vi "Create Dir in FTP if Not Exist.vi"(8 "error in (no error)":errorcluster, 10 "dir":string, 11 "FTPProtocol in":refnum<class "FTPProtocol.lvclass">) -> (0 "error out":errorcluster, 3 "FTPProtocol out":refnum<class "FTPProtocol.lvclass">)   [LabVIEW 2020, in "CSM-FileSync.lvlib" / "FTPProtocol.lvclass"]
uses:
  FTPProtocol.lvclass
  FTPProtocol.lvclass/FTPProtocol.ctl
  Read FTP.vi
  FTP Toolkit/FTP Class/FTP.lvclass
  <userlib>/_NEVSTOP/Communicable State Machine(CSM)/_Shared/CSM Shared.lvlib
  <userlib>/_NEVSTOP/Communicable State Machine(CSM)/Communicable State Machine.lvlib
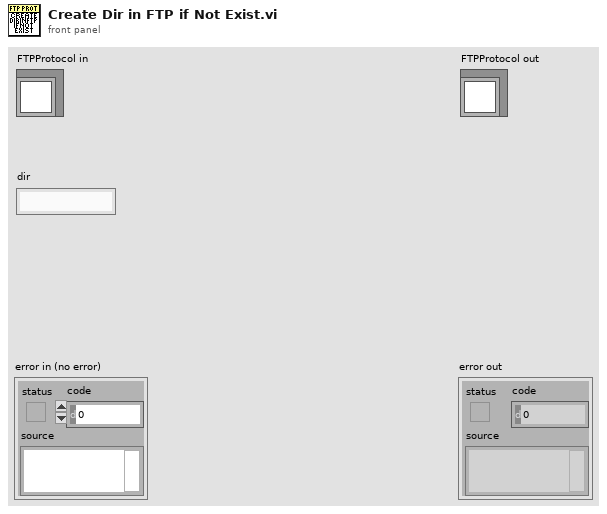
[diagram p1: front panel]
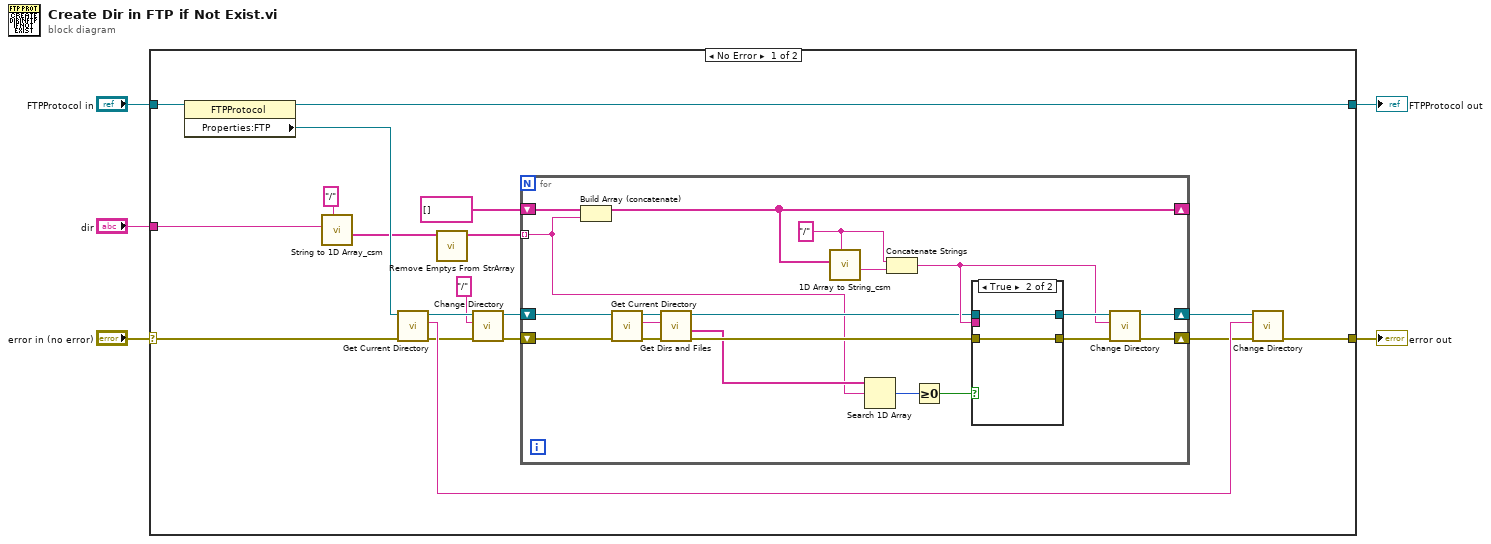
[diagram p0: block diagram]
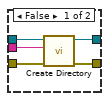
[diagram p2: hidden frame]
diagram:
  n1 = case shown="No Error" "error in (no error)" {
    selector: "error in (no error)" -> [w13 w52]
    tunnel: [w16 w52] -> w4
    tunnel: [w22 w51] -> w2
    tunnel: "FTPProtocol in" -> [w23 w51]
    tunnel: "dir" -> [w20 _]
    frame No Error {
      n2 = property class="FTPProtocol"(reference=w23) -> (reference out=w22:refnum<class "FTPProtocol.lvclass">, "Properties:FTP"=w15:refnum<class "FTP.lvclass">)  [unwired: 1 in, 1 out]
      n3 = call <userlib>:"String to 1D Array_csm.vi"("delimiter (Tab)"="/", "string"=w20) -> ("Array of Strings"=w11:string[])  [unwired: 9 in]
      n4 = call "Get Current Directory.vi"("error in (no error)"=w13, "FTP in"=w15) -> ("error out"=w9:errorcluster, "Current Directory"=w18:string, "FTP out"=w10:refnum<class "FTP.lvclass">)  [unwired: 7 in]
      n5 = call <userlib>:"Remove Emptys From StrArray.vi"("Array In"=w11) -> ("Array Out"=w12:string[])  [unwired: 10 in]
      n6 = call "Change Directory.vi"("error in (no error)"=w9, "RemoteDirectory"="/" ("delimiter (Tab)"), "FTP in"=w10) -> ("error out"=w7:errorcluster, "FTP out"=w8:refnum<class "FTP.lvclass">)  [unwired: 7 in]
      n7 = for {
        shift-right: [w38] -> w19
        shift-left: w8 -> [w33]
        shift-right: [w39] -> w17
        shift-left: w7 -> [w32]
        tunnel: w12 -> [w24] mode=indexing
        shift-right: [w42] -> _
        shift-left: string[] [] ("delimiter (Tab)") -> [w43]
        w36 = "/" ("delimiter (Tab)")
        n8 = Build Array (concatenate)(w43, w24) -> (w42:string[])
        n9 = call "Get Current Directory.vi"("error in (no error)"=w32, "FTP in"=w33) -> ("error out"=w31:errorcluster, "Current Directory"=w29:string, "FTP out"=w30:refnum<class "FTP.lvclass">)  [unwired: 7 in]
        n10 = call "Get Dirs and Files.vi"("error in (no error)"=w31, "RemoteDirectory"=w29, "FTP in"=w30) -> ("error out"=w34:errorcluster, "Dirs"=w25:string[], "FTP out"=w35:refnum<class "FTP.lvclass">)  [unwired: 5 in, 1 out]
        n11 = call <userlib>:"1D Array to String_csm.vi"("delimiter (Tab)"=w36, "Array of Strings"=w42) -> ("delimited string"=w28:string)  [unwired: 9 in]
        n12 = Search 1D Array(1D array=w25, element=w24) -> (index of element=w27:i32)  [unwired: 1 in]
        n13 = Concatenate Strings(w36, w28) -> (w37:string)
        n14 = Greater Or Equal To 0?(x=w27) -> (x >= 0?=w26:bool)
        n15 = case shown="True" w26 {
          tunnel: [w48 w50] -> w41
          tunnel: [w47 w49] -> w40
          tunnel: w37 -> [w46 _]
          tunnel: w35 -> [w45 w50]
          tunnel: w34 -> [w44 w49]
          frame False {
            n16 = call "Create Directory.vi"("error in (no error)"=w44, "Remote Directory"=w46, "FTP in"=w45) -> ("error out"=w47:errorcluster, "FTP out"=w48:refnum<class "FTP.lvclass">)  [unwired: 7 in]
          }
          frame True {
          }
        }
        n17 = call "Change Directory.vi"("error in (no error)"=w40, "RemoteDirectory"=w37, "FTP in"=w41) -> ("error out"=w39:errorcluster, "FTP out"=w38:refnum<class "FTP.lvclass">)  [unwired: 7 in]
      }
      n18 = call "Change Directory.vi"("error in (no error)"=w17, "RemoteDirectory"=w18, "FTP in"=w19) -> ("error out"=w16:errorcluster)  [unwired: 7 in, 1 out]
    }
    frame Error {
    }
  }
  "error out" <- w4
  "FTPProtocol out" <- w2
